vi "Timing Error Info.vi"(11 "error":T1) -> (3 "error info":cluster{"code":i32, "description":string})   [LabVIEW 2017, in "DSF Core.lvlib" / "Timing.lvclass"]
uses:
  Timing.lvclass
  Errors.ctl
  Constants/Base Error Code.vi
  DSF Core.lvlib
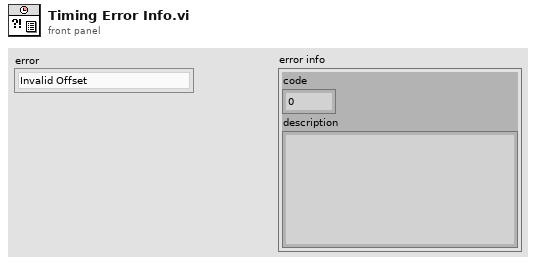
[diagram p1: front panel]
types:
  T1 = typedef "DSF Core.lvlib/Timing.lvclass/Errors.ctl" = enum16{"Invalid Offset", "Invalid Priority"}
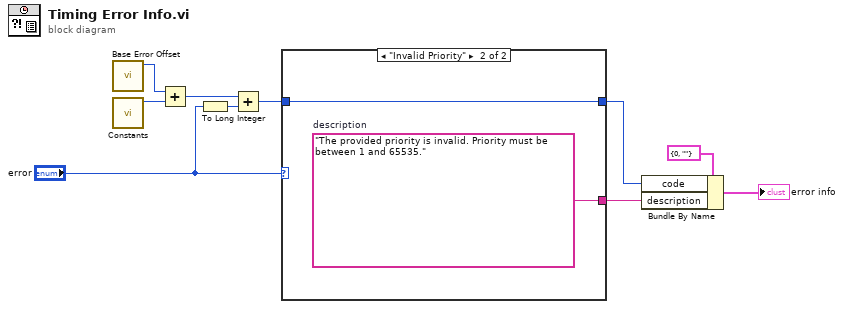
[diagram p0: block diagram]
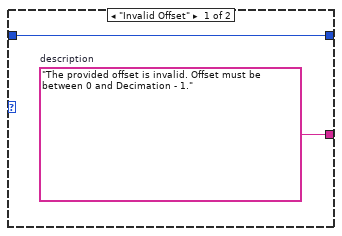
[diagram p2: hidden frame]
diagram:
  n1 = call "Base Error Offset.vi"() -> ("base error offset"=w2:i32)  [unwired: 11 in]
  n2 = call-poly "Constants.vi"() -> ("base error code"=w10:i32)  [unwired: 11 in]
  n3 = Add(x=w2, y=w10) -> (x+y=w6:i32)
  n4 = To Long Integer(number="error") -> (32bit integer=w9:i32)
  n5 = Add(x=w6, y=w9) -> (x+y=w5:i32)
  n6 = case shown="\"Invalid Priority\"" "error" {
    tunnel: [w12 w14] -> w7
    tunnel: w5 -> [w11 w13]
    tunnel: [w11 w13] -> w4
    frame "Invalid Offset" {
      w12 = "The provided offset is invalid. Offset must be between 0 and Decimation - 1."  # description
    }
    frame "Invalid Priority" {
      w14 = "The provided priority is invalid. Priority must be between 1 and 65535."  # description
    }
  }
  n7 = Bundle By Name(cluster=cluster{"code":i32, "description":string} {"code"=0, "description"=""}, "code"=w4, "description"=w7) -> (→"error info":cluster{"code":i32, "description":string})
